vi "TC10 Status.vi"(8 "error in (no error)":errorcluster, 9 "Interface Name":refnum<k21>, 11 "XNET Session":refnum<k21>) -> (0 "error out":errorcluster, 1 "TC10 Mode":bool, 3 "XNET Session Out":refnum<k21>)   [LabVIEW 2025, in "Automotive Ethernet Bus Monitor UI.lvlib"]
uses:
  Automotive Ethernet Bus Monitor UI.lvlib
  <vilib>/xnet/xnet.llb/XNET Create Session (Frame Input Stream).vi
  <resource>/objmgr/xnet.rc
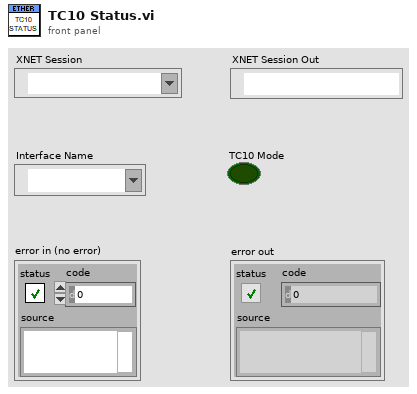
[diagram p1: front panel]
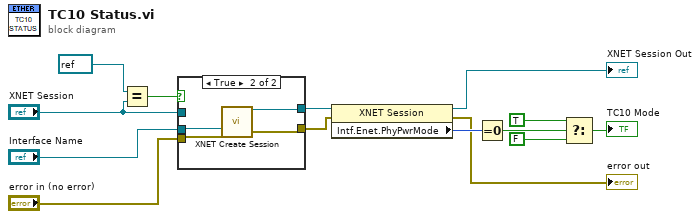
[diagram p0: block diagram]
diagram:
  n1 = Equal?(x=refnum<k21> refnum ("XNET Session"), y="XNET Session") -> (x = y?=w11:bool)
  n2 = case shown="True" w11 {
    tunnel: [w15 w18] -> w7
    tunnel: [_ w19] -> w8
    tunnel: "Interface Name" -> [_ w17]
    tunnel: "XNET Session" -> [w15 _]
    tunnel: "error in (no error)" -> [_ w16]
    frame False {
    }
    frame True {
      n3 = call-poly <vilib>:"XNET Create Session.vi"("interface"=w17, "error in (no error)"=w16) -> ("session out"=w18:refnum<k21>, "error out"=w19:errorcluster)  [unwired: 12 in]
    }
  }
  n4 = property class="XNET Session"(reference=w7, error in=w8) -> (reference out=→"XNET Session Out":refnum<k21>, error out=→"error out":errorcluster, "Intf.Enet.PhyPwrMode"=w10:u32)
  n5 = Equal To 0?(x=w10) -> (x = 0?=w9:bool)
  n6 = Select(t=TRUE, s=w9, f=FALSE) -> (s? t:f=→"TC10 Mode":bool)
